vi "Keyence_写入单个线圈数据.vi"(0 "Keyence ID In":refnum<k5>, 1 "Delay Time (s)":dbl=1.0 caption="延迟时间(s)", 5 "软元件编号":string, 9 "应用模式":string(combo), 11 "错误输入（无错误）":errorcluster) -> (4 "Keyence ID Out":refnum<k5>, 10 "状态":bool, 15 "错误输出":errorcluster)   [LabVIEW 2017]
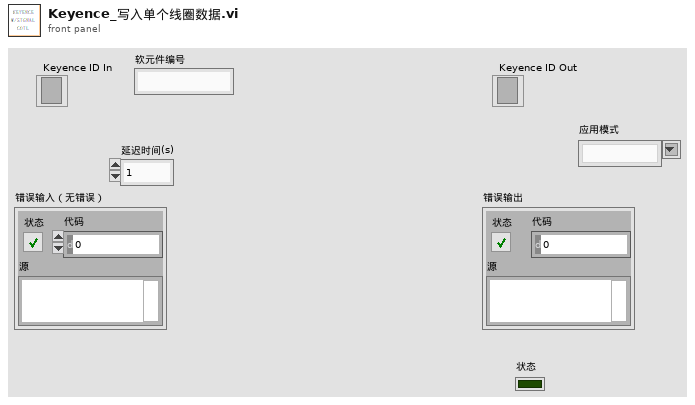
[diagram p1: front panel]
types:
  T1 = enum16{"Standard", "Buffered", "CRLF", "Immediate"}
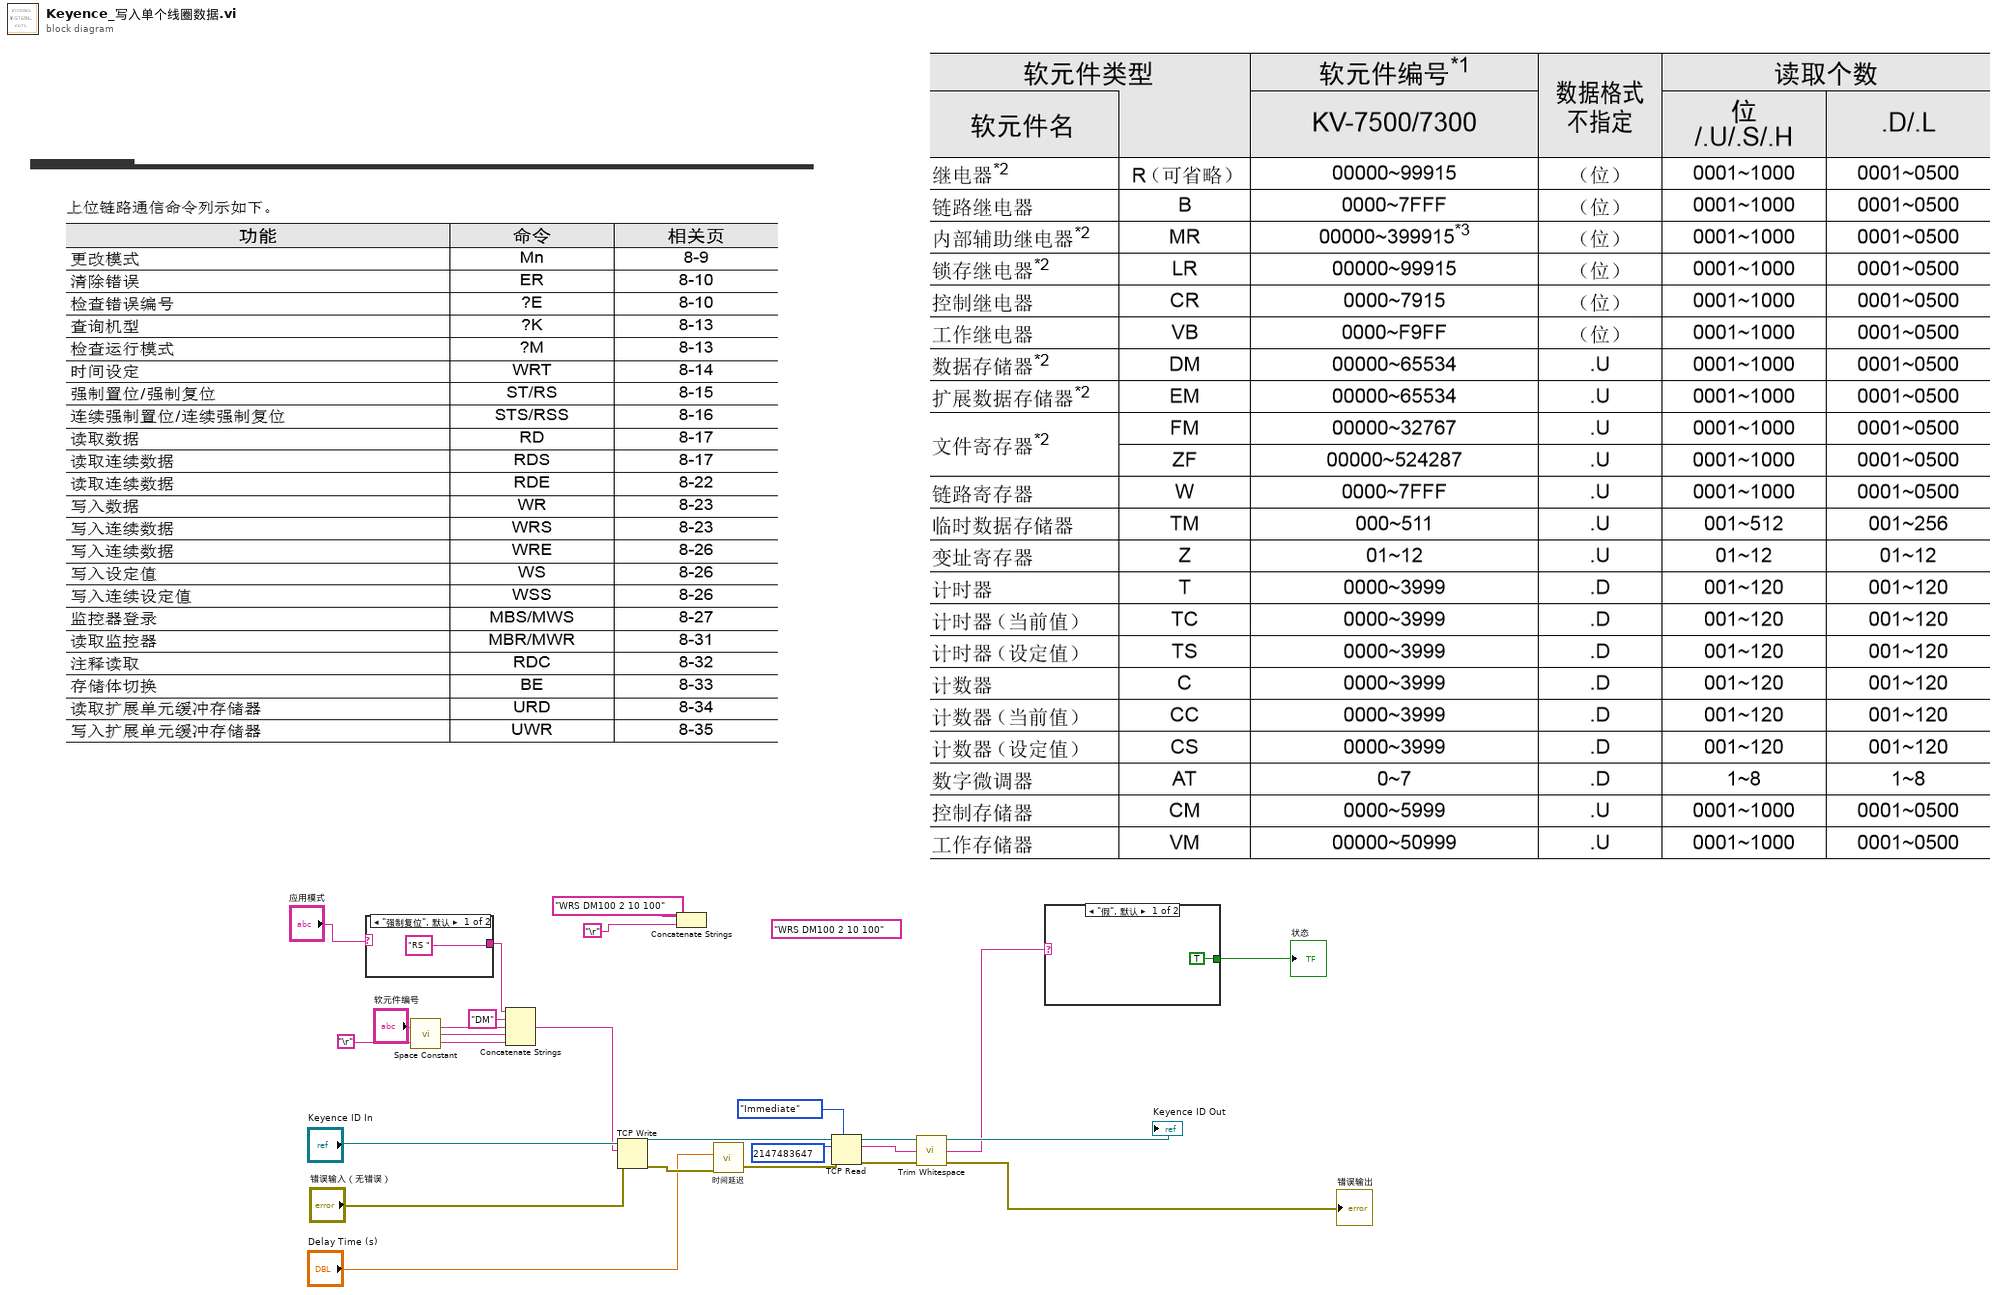
[diagram p0: block diagram]
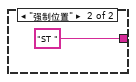
[diagram p2: hidden frame]
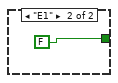
[diagram p3: hidden frame]
diagram:
  (unwired) "WRS DM100 2 10 100"
  n1 = case shown="\"强制复位\", 默认" "应用模式" {
    tunnel: ["RS " "ST "] -> w1
    frame "强制复位", Default {
    }
    frame "强制位置" {
    }
  }
  n2 = call <vilib>:"Space Constant.vi"() -> ("String"=w10:string)
  n3 = Concatenate Strings(w1, "DM" ("字符串"), "软元件编号", w10, "\r") -> (w8:string)
  n4 = TCP Write(connection ID="Keyence ID In", data in=w8, error in (no error)="错误输入（无错误）") -> (connection ID out=w20:refnum<k5>, error out=w19:errorcluster)  [unwired: 1 in, 1 out]
  n5 = Concatenate Strings("WRS DM100 2 10 100", "\r") -> ()  [unwired: 1 out]
  n6 = call "时间延迟"("error in (no error)"=w19, "Delay Time (s)"="Delay Time (s)") -> ("error out"=w14:errorcluster)  [unwired: 9 in]
  n7 = TCP Read(connection ID=w20, bytes to read=2147483647 ("读取的字节"), error in (no error)=w14, 7:T1."Immediate" ("模式（标准）")) -> (connection ID out=→"Keyence ID Out":refnum<k5>, data out=w5:string, error out=→"错误输出":errorcluster)  [unwired: 1 in]
  n8 = call <vilib>:"Trim Whitespace.vi"("string"=w5) -> ("trimmed string"=w4:string)  [unwired: 1 in]
  n9 = case shown="\"假\", 默认" w4 {
    tunnel: [TRUE FALSE] -> w3
    frame "假", Default {
    }
    frame "E1" {
    }
  }
  "状态" <- w3
